vi "Valid Replacement Target.vi"(8 "error in (no error)":errorcluster, 11 "object reference in":refnum<vi>) -> (0 "error out":errorcluster, 1 "missing path":path, 2 "missing name":string, 3 "object reference out":refnum<vi>, 4 "valid replacement target":bool)   [LabVIEW 2021, in "MeasurementService Editor.lvlib"]
uses:
  MeasurementService Editor.lvlib
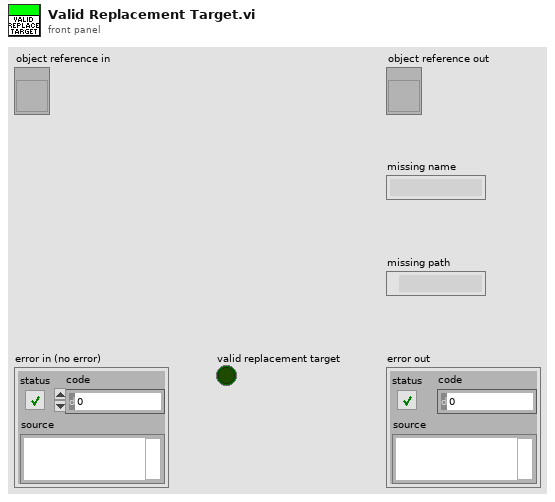
[diagram p1: front panel]
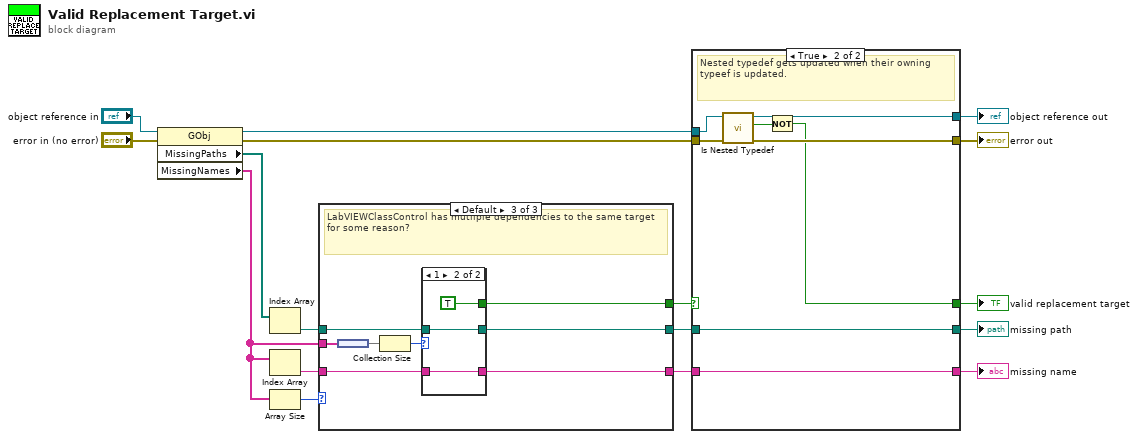
[diagram p0: block diagram]
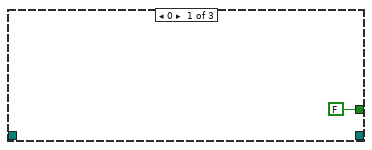
[diagram p3: hidden frame]
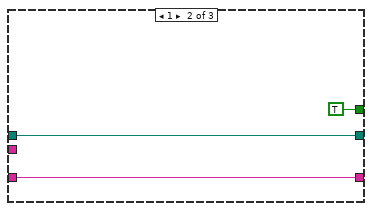
[diagram p4: hidden frame]
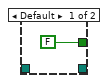
[diagram p5: hidden frame]
diagram:
  n1 = property class="GObj"(reference="object reference in", error in="error in (no error)") -> (reference out=w2:refnum<vi>, error out=w4:errorcluster, "MissingPaths"=w13:path[], "MissingNames"=w12:string[])
  n2 = Index Array(array=w13) -> (element=w15:path)  [unwired: 1 in]
  n3 = Index Array(array=w12) -> (element=w16:string)  [unwired: 1 in]
  n4 = Array Size(array=w12) -> (size(s)=w17:i32)
  n5 = case shown="Default" w17 {
    tunnel: w16 -> [_ w21 w24]
    tunnel: w15 -> [_ w20 w22]
    tunnel: [_ w21 w25] -> w7
    tunnel: [_ w20 w23] -> w8
    tunnel: [FALSE TRUE w26] -> w10
    tunnel: w12 -> [_ _ w28]
    frame 0 {
    }
    frame 1 {
    }
    frame Default {
      # "LabVIEWClassControl has mutliple dependencies to the same target for some reason?"
      n6 = node(w28) -> (w29:set{string[]})
      n7 = Collection Size(1:w29) -> (0:w27:i32)
      n8 = case shown="1" w27 {
        tunnel: [FALSE TRUE] -> w26
        tunnel: [_ w32] -> w25
        tunnel: w24 -> [_ w32]
        tunnel: [_ w31] -> w23
        tunnel: w22 -> [_ w31]
        frame Default {
        }
        frame 1 {
        }
      }
    }
  }
  n9 = case shown="True" w10 {
    selector: w10 -> [w36 _]
    tunnel: [w36 w37] -> w9
    tunnel: w8 -> [_ w44]
    tunnel: w7 -> [_ w43]
    tunnel: [_ w44] -> w6
    tunnel: [_ w43] -> w5
    tunnel: w4 -> [w35 w42]
    tunnel: [w35 w41] -> w3
    tunnel: w2 -> [w34 w40]
    tunnel: [w34 w39] -> w1
    frame False {
    }
    frame True {
      # "Nested typedef gets updated when their owning typeef is updated."
      n10 = call "Is Nested Typedef.vi"("error in (no error)"=w42, "object reference in"=w40) -> ("error out"=w41:errorcluster, "is nested typedef?"=w38:bool, "object reference out"=w39:refnum<vi>)  [unwired: 7 in]
      n11 = Not(x=w38) -> (.not. x?=w37:bool)
    }
  }
  "missing path" <- w6
  "missing name" <- w5
  "error out" <- w3
  "valid replacement target" <- w9
  "object reference out" <- w1
